vi "DI Read Body.vi"(6 "error in":errorcluster, 9 "Channel":tag) -> (0 "error out":errorcluster, 2 "data":bool)   [LabVIEW 2015, in "DAQ.lvlib"]
uses:
  DAQ.lvlib
  <vilib>/DAQmx/create/channels.llb/DAQmx Create Channel (AI-Voltage-Basic).vi
  <vilib>/DAQmx/read.llb/DAQmx Read (Analog DBL 1Chan 1Samp).vi
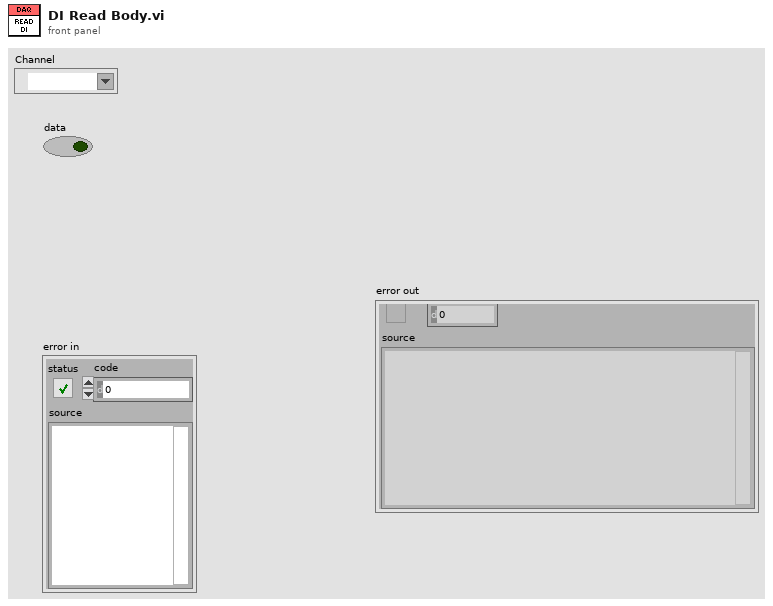
[diagram p1: front panel]
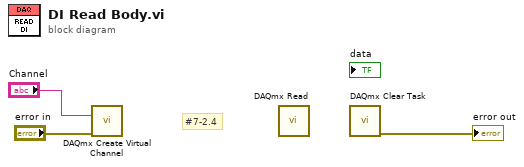
[diagram p0: block diagram]
diagram:
  # "#7-2.4"
  n1 = call-poly <vilib>:"DAQmx Create Virtual Channel.vi"("physical channels"="Channel", "error in"="error in") -> ()  [unwired: 12 in, 2 out]
  n2 = call-poly <vilib>:"DAQmx Read.vi"() -> ()  [unwired: 13 in, 3 out]
  n3 = call <vilib>:"DAQmx Clear Task.vi"() -> ("error out"=→"error out":errorcluster)  [unwired: 15 in]
